vi "Read Configuration File.vi"(8 "error in (no error)":errorcluster, 11 "Inst.Framework-Template in":refnum<class "Inst.Framework-Template.lvclass">) -> (0 "error out":errorcluster, 3 "Inst.Framework-Template out":refnum<class "Inst.Framework-Template.lvclass">)   [LabVIEW 2019, in "Inst.Framework-Template.lvclass"]
uses:
  Inst.Framework-Template.lvclass
  C:/Program Files (x86)/National Instruments/LabVIEW 2019/user.lib/LevyLab/Instrument Framework/SMOs/Instrument/Instrument.lvclass
  <userlib>/LevyLab/Instrument Framework/SMOs/Instrument/Instrument.lvclass/Instrument.ctl
  <userlib>/LevyLab/Instrument Framework/SMOs/Configuration/Configuration.lvclass/Configuration.ctl
  Inst.Framework-Template.lvclass/Inst.Framework-Template.ctl
  <userlib>/LevyLab/Instrument Framework/SMOs/Configuration/Write Section.vi
  <userlib>/LevyLab/Instrument Framework/SMOs/Instrument/Instrument.lvclass
  C:/Program Files (x86)/National Instruments/LabVIEW 2019/vi.lib/JKI/JKI SMO/SMO/SMO.lvclass
  <vilib>/JKI/JKI SMO/SMO/Protected/ThisLevelClassName.vi
  <userlib>/LevyLab/Instrument Framework/Instrument Types/VSource/Instrument.VSource.lvclass
  <userlib>/LevyLab/Instrument Framework/SMOs/Configuration/Configuration.lvclass
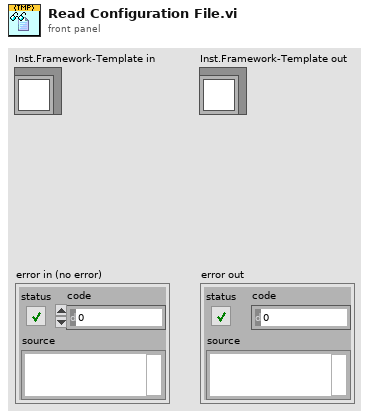
[diagram p1: front panel]
types:
  T1 = typedef "Inst.Framework-Template.lvclass/Inst.Framework-Template.Configuration--Cluster.ctl" = cluster{"Example Setting 1":dbl, "Example Setting 2":dbl, "Example Setting 3":string}
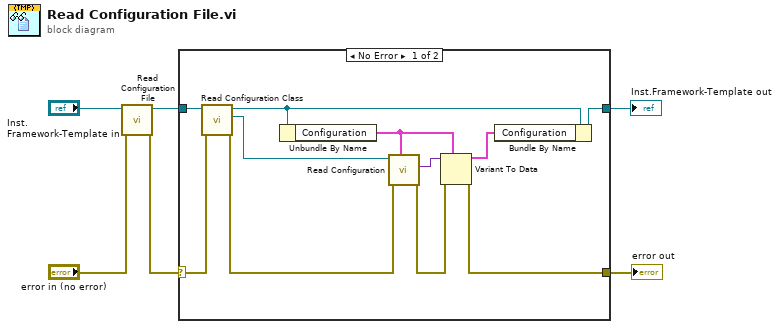
[diagram p0: block diagram]
diagram:
  n1 = call-parent "Read Configuration File.vi"("error in (no error)"="error in (no error)", "Instrument in"="Inst.Framework-Template in") -> ("error out"=w1:errorcluster, "Instrument out"=w3:refnum<class "Inst.Framework-Template.lvclass">)  [unwired: 8 in]
  n2 = case shown="No Error" w1 {
    selector: w1 -> [w14 w19]
    tunnel: w3 -> [w16 w18]
    tunnel: [w10 w18] -> w6
    tunnel: [w15 w19] -> w5
    frame No Error {
      n3 = call <userlib>:"Read Configuration Class.vi"("error in (no error)"=w14, "Instrument in"=w16) -> ("error out"=w11:errorcluster, "Configuration"=w9:refnum<class "Configuration.lvclass">, "Instrument out"=w8:refnum<class "Inst.Framework-Template.lvclass">)  [unwired: 7 in]
      n4 = Unbundle By Name(w8) -> ("Configuration"=w13:T1)
      n5 = call <userlib>:"Read Configuration.vi"("INI Fomatted Cluster Type"=w13, "error in (no error)"=w11, "Configuration in"=w9) -> ("error out"=w17:errorcluster, "Configuration"=w12:variant)  [unwired: 6 in, 1 out]
      n6 = Variant To Data(error in=w17, type=w13, Variant=w12) -> (data=w7:T1, error out=w15:errorcluster)
      n7 = Bundle By Name(cluster=w8, "Configuration"=w7) -> (w10:refnum<class "Inst.Framework-Template.lvclass">)
    }
    frame Error {
    }
  }
  "Inst.Framework-Template out" <- w6
  "error out" <- w5
